vi "Digital Input Single Read.vi"() -> ()   [LabVIEW 2009, in "MicroDAQ.lvlib"]
uses:
  <instrlib>/MicroDAQ/MicroDAQ.lvlib
  <instrlib>/MicroDAQ/Tools/Digital IO channels.ctl
  <instrlib>/MicroDAQ/Channel/Digital Input/Read NPorts 1Sampe 1D U8.vi
  <instrlib>/MicroDAQ/Channel/Digital Input/Digital Input.lvclass
panel:
  out "data":u8[](array[numeric]) format="%08b"
  in  "Lines":T1[](array[typedef])=[1] items=["DIO1...8"=1, "DIO9...16"=2, "DIO17...24"=3, "DIO25...32"=4]
  in  "IP address":string="10.10.1.1"
  # "Device settings"
  # "Channel Settings"
  # "Input"
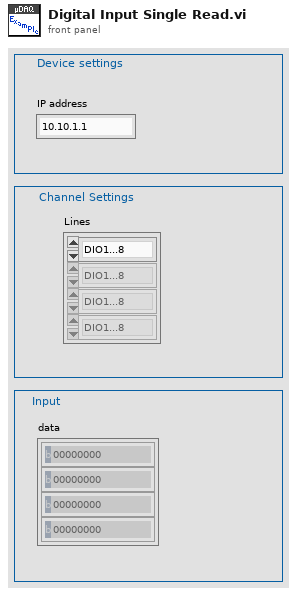
[diagram p1: front panel]
types:
  T1 = typedef "MicroDAQ.lvlib/Digital IO channels.ctl" = u8
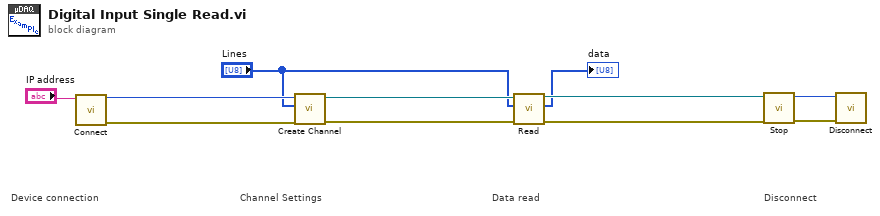
[diagram p0: block diagram]
diagram:
  # "Disconnect"
  # "Data read"
  # "Channel Settings"
  # "Device connection"
  n1 = call <instrlib>:"Connect.vi"("IP address"="IP address") -> ("error out"=w11:errorcluster, "connection ID"=w10:i32)  [unwired: 9 in]
  n2 = call-poly <instrlib>:"Create Channel.vi"("error in (no error)"=w11, "Lines"="Lines", "Connection ID"=w10) -> ("error out"=w7:errorcluster, "MicroDAQ.lvlib:Digital Input.lvclass"=w8:refnum<class "Digital Input.lvclass">)  [unwired: 7 in]
  n3 = call-poly <instrlib>:"Read.vi"("error in (no error)"=w7, "Ports (Banks)"="Lines", "MicroDAQ.lvlib:Digital Input.lvclass"=w8) -> ("error out"=w4:errorcluster, "data"=→"data":u8[], "MicroDAQ.lvlib:Digital Input.lvclass out"=w5:refnum<class "Digital Input.lvclass">)  [unwired: 6 in]
  n4 = call-dynamic "Stop.vi"("error in (no error)"=w4, "Task in"=w5) -> ("error out"=w3:errorcluster, "connection ID"=w2:i32)  [unwired: 8 in]
  n5 = call <instrlib>:"Disconnect.vi"("error in (no error)"=w3, "connection ID"=w2) -> ()  [unwired: 9 in, 1 out]
